vi "ReadSensorValues.vi"(10 "VISA resource name":refnum<visa-resource-name>, 11 "Sensor type":T1=enum."CAB 300-C SP3 (CAN)") -> ()   [LabVIEW 2012]
uses:
  <vilib>/nican/nicantsk.llb/CAN Interface.ctl
  SensorTypes.ctl
  SensorStates.ctl
  <vilib>/nican/nicantsk.llb/CAN Task Reference.ctl
  <vilib>/nican/nicantsk.llb/CAN Mode.ctl
  <vilib>/Analysis/3filter.llb/Filter Passband Type.ctl
  globalVariables.vi
  <vilib>/nican/nicantsk.llb/CAN Read Multi Chan Single Samp 1D Dbl.vi
  <vilib>/ptbypt/NI_PtbyPt.lvlib
  <vilib>/Analysis/NI_AALBase.lvlib
panel:
  out "Waveform Chart":dbl[](graph)
  out "Filtered current":dbl format="%.2f"
  in  "Cancel Measurement":bool
  out "new data":bool
  out "running":bool
  out "Sample number":i32
  in  "Interface":T2 items=["CAN0"=0, "CAN1"=1, "CAN2"=2, "CAN3"=3, "CAN4"=4, "CAN5"=5, "CAN6"=6, "CAN7"=7, "CAN8"=8, "CAN9"=9, "CAN10"=10, "CAN11"=11, "CAN12"=12, "CAN13"=13, "CAN14"=14, "CAN15"=15, "CAN16"=16, "CAN17"=17, "CAN18"=18, "CAN19"=19, "CAN20"=20, "CAN21"=21, "CAN22"=22, "CAN23"=23, "CAN24"=24, "CAN25"=25, "CAN26"=26, "CAN27"=27, "CAN28"=28, "CAN29"=29, "CAN30"=30, "CAN31"=31, "CAN32"=32, "CAN33"=33, "CAN34"=34, "CAN35"=35, "CAN36"=36, "CAN37"=37, "CAN38"=38, "CAN39"=39, "CAN40"=40, "CAN41"=41, "CAN42"=42, "CAN43"=43, "CAN44"=44, "CAN45"=45, "CAN46"=46, "CAN47"=47, "CAN48"=48, "CAN49"=49, "CAN50"=50, "CAN51"=51, "CAN52"=52, "CAN53"=53, "CAN54"=54, "CAN55"=55, "CAN56"=56, "CAN57"=57, "CAN58"=58, "CAN59"=59, "CAN60"=60, "CAN61"=61, "CAN62"=62, "CAN63"=63, "MAX default"=64, "CAN256 (Virtual)"=256, "CAN257 (Virtual)"=257]
  out "current":dbl format="%^#_5e"
  out "Error Flag":bool
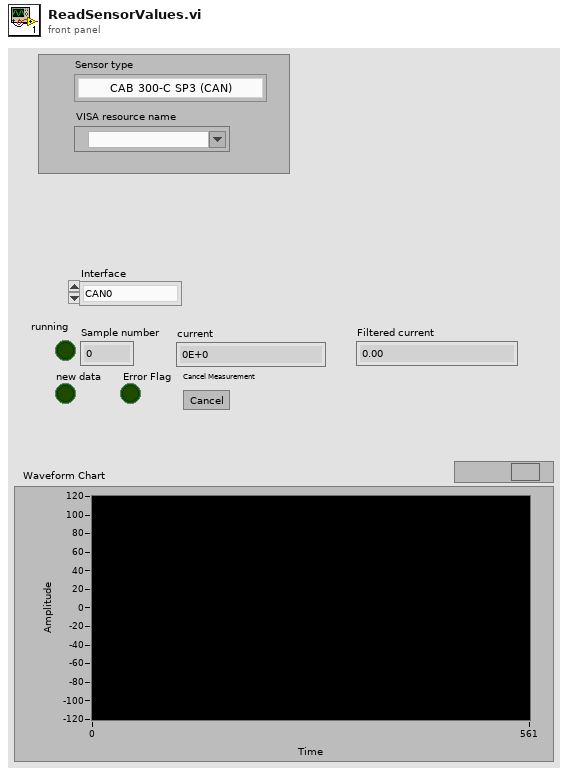
[diagram p1: front panel]
types:
  T1 = typedef "SensorTypes.ctl" = enum16{"ITL 900 (Analogue)", "CAB 300-C SP3 (CAN)", "xyz TODO (PWM)", "xyz TODO (LIN)", "xyz TODO (Analogue)"}
  T2 = typedef "CAN Interface.ctl" = u16
  T3 = typedef "SensorStates.ctl" = enum16{"init", "measure", "terminate"}
  T4 = typedef "CAN Task Reference.ctl" = u32
  T5 = typedef "NI_AALBase.lvlib/Filter Passband Type.ctl" = enum32{"Lowpass", "Highpass", "Bandpass", "Bandstop"}
  T6 = typedef "CAN Mode.ctl" = u16
  T7 = typedef "TimeValue.ctl" = cluster{"Time of measurement":timestamp, "Current value":dbl}
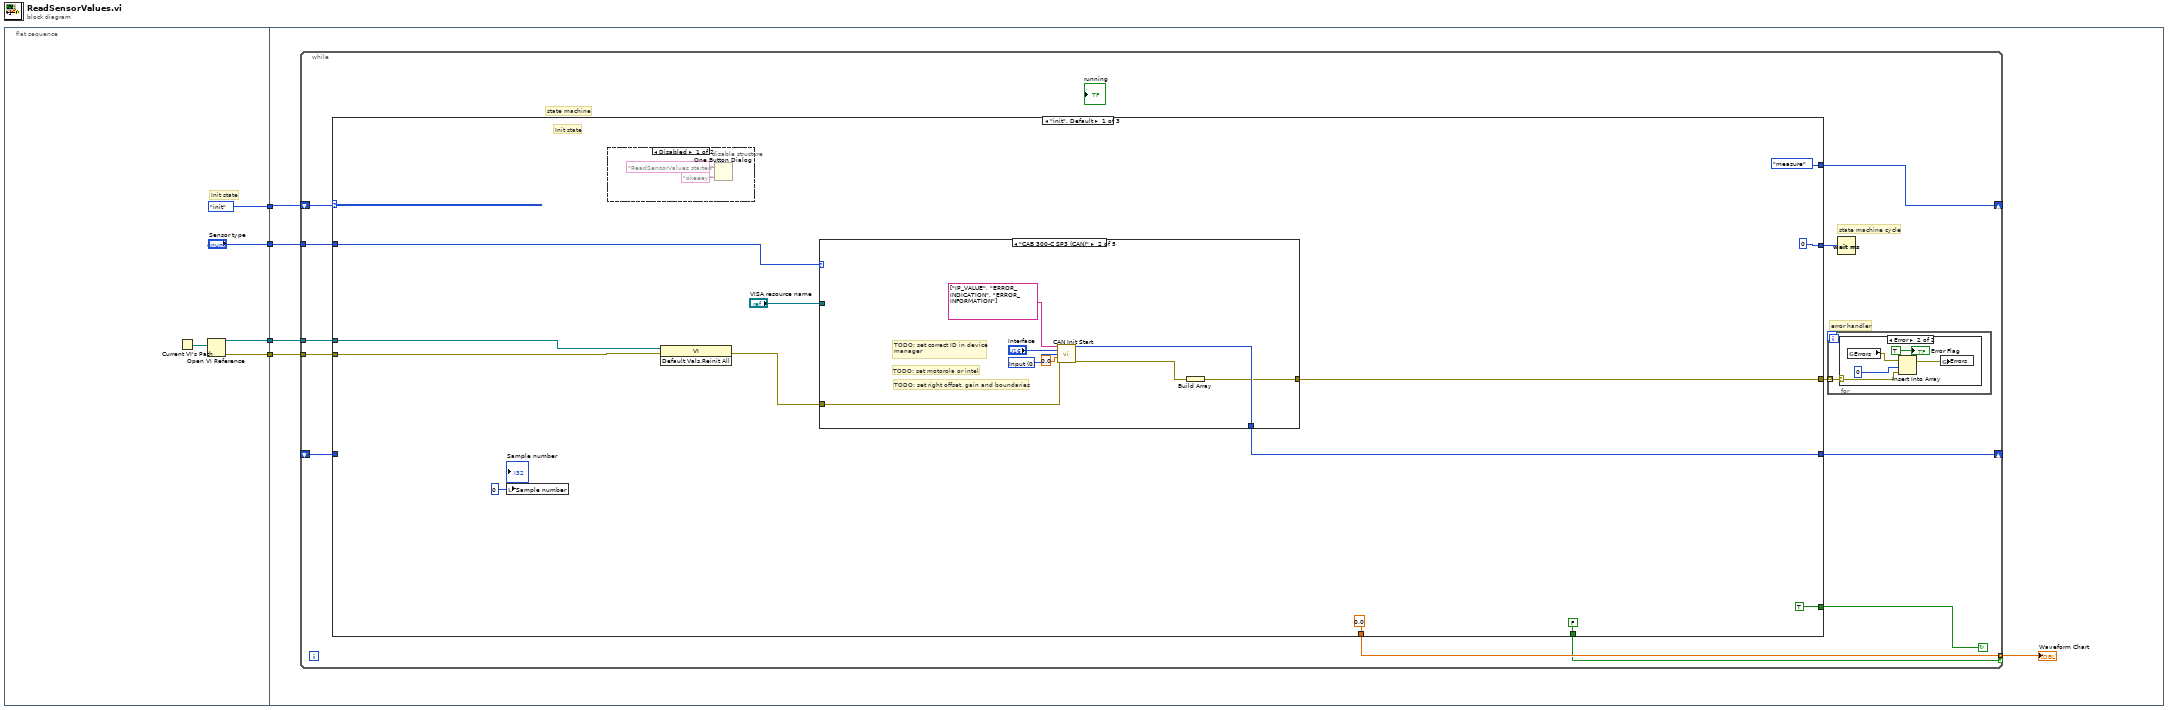
[diagram p0: block diagram]
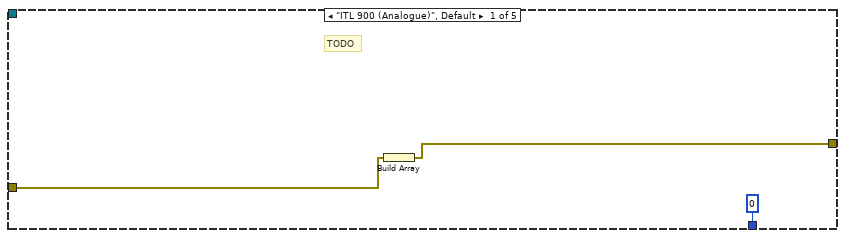
[diagram p4: hidden frame]
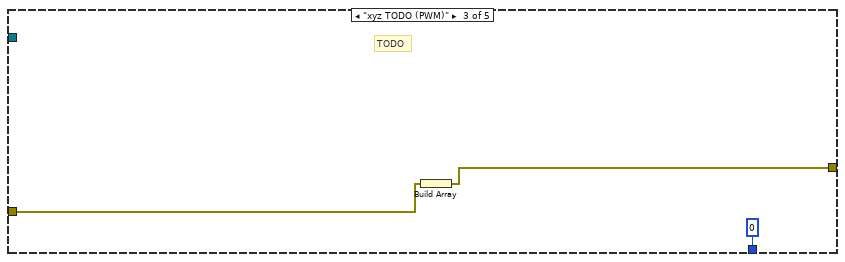
[diagram p5: hidden frame]
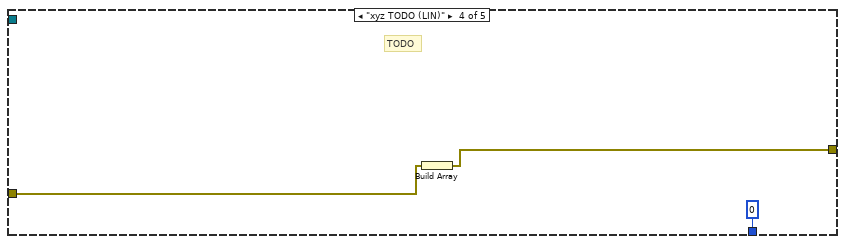
[diagram p6: hidden frame]
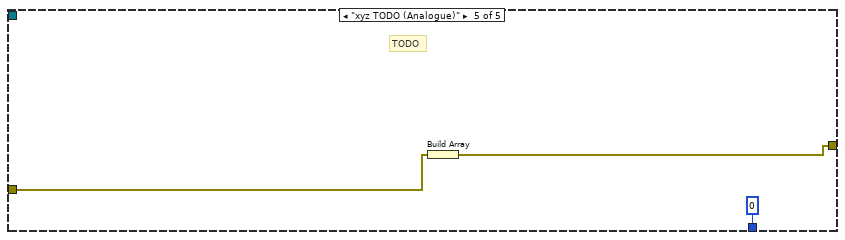
[diagram p7: hidden frame]
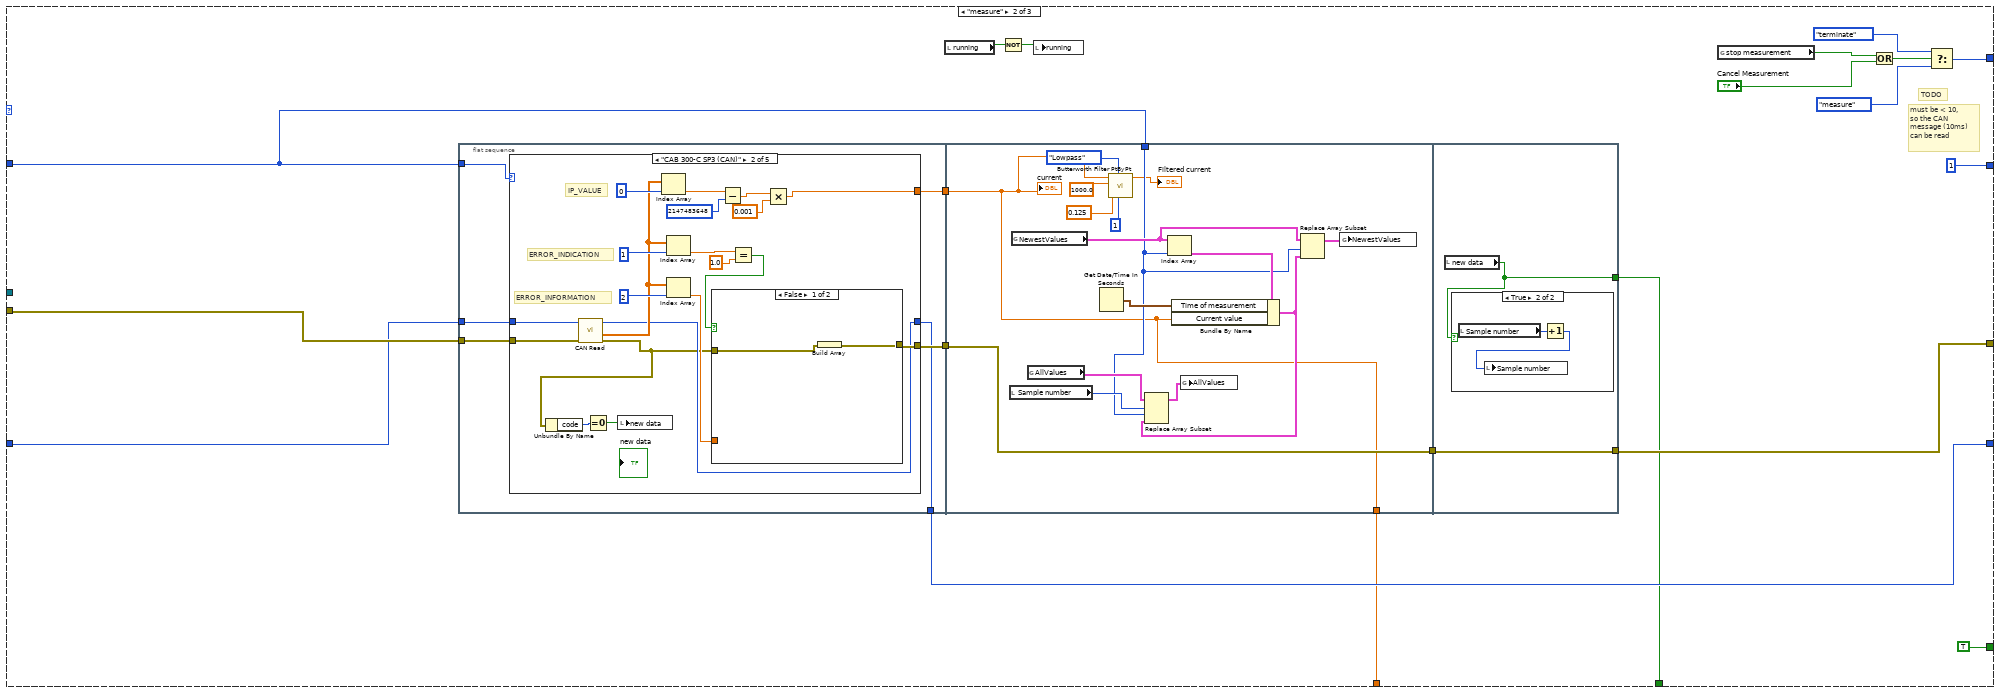
[diagram p8: hidden frame]
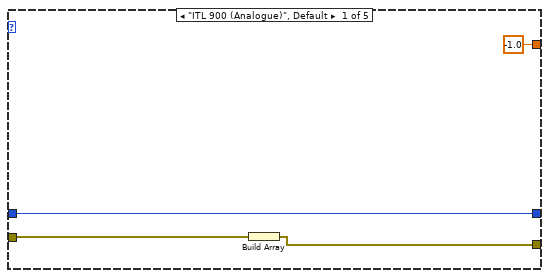
[diagram p9: hidden frame]
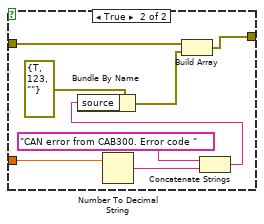
[diagram p10: hidden frame]
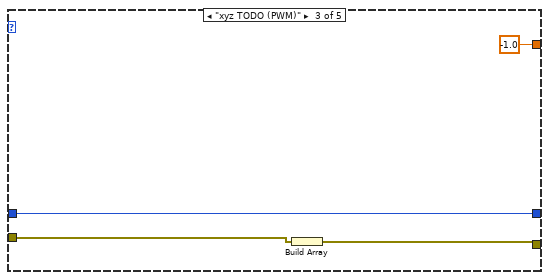
[diagram p11: hidden frame]
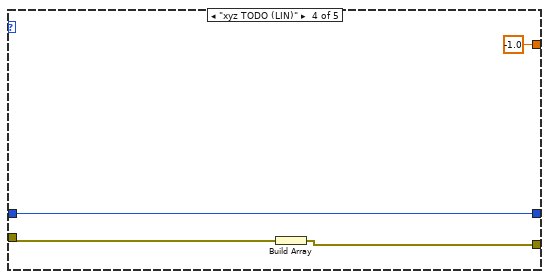
[diagram p12: hidden frame]
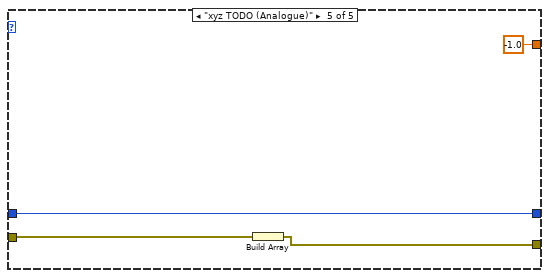
[diagram p13: hidden frame]
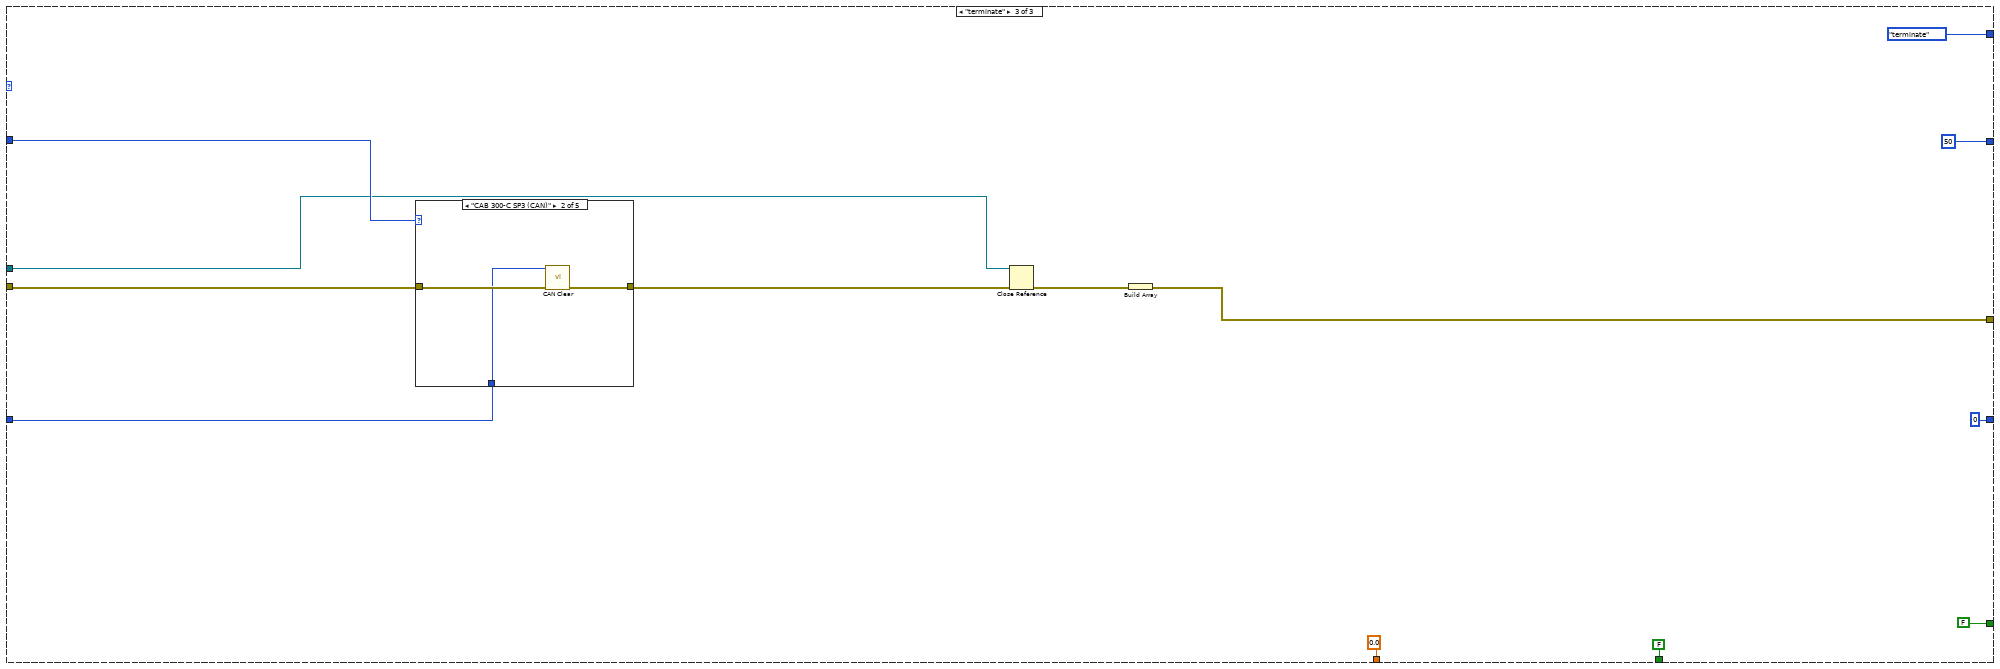
[diagram p15: hidden frame]
diagram:
  n1 = flat-sequence {
    tunnel: [SensorStates."init" ("States IEEE-488")] -> w4
    tunnel: [w9] -> w3
    tunnel: [w8] -> w2
    tunnel: ["Sensor type"] -> w1
    tunnel: w4 -> [w12]
    tunnel: w3 -> [w14]
    tunnel: w2 -> [w13]
    tunnel: w1 -> [w11]
    frame #0 {
      # "Init state"
      n2 = Current VI's Path() -> (path=w7:path)
      n3 = Open VI Reference(vi path=w7) -> (vi reference=w9:refnum<vi>, error out=w8:errorcluster)  [unwired: 2 in, 3 out]
    }
    frame #1 {
      n4 = while {
        tunnel: w14 -> [w25]
        tunnel: w13 -> [w24]
        shift-right: [w22] -> _
        shift-left: w12 -> [w23]
        shift-right: [w21] -> _
        shift-left: _ -> [w20]
        tunnel: w11 -> [w18]
        tunnel: [w16] -> w10 mode=indexing if=w15
        stop <- w17 continue-if-true
        # "state machine"
        # "error handler"
        # "state machine cycle"
        n5 = case shown="\"init\", Default" w23 {
          tunnel: [u32 0 ("milliseconds to wait") u32 1 ("milliseconds to wait") u32 50 ("milliseconds to wait")] -> w26
          tunnel: w25 -> [w43 _ w164]
          tunnel: w24 -> [w44 w83 w169]
          tunnel: [SensorStates."measure" ("States IEEE-488") w84 SensorStates."terminate" ("States IEEE-488")] -> w22
          tunnel: [w41 w73 T4 0 ("task reference out")] -> w21
          tunnel: w20 -> [_ w74 w168]
          tunnel: [w39 w75 w167] -> w19
          tunnel: w18 -> [w37 w79 w166]
          tunnel: [TRUE TRUE FALSE] -> w17
          tunnel: [0.0 ("Sample") w69 0.0 ("Sample")] -> w16
          tunnel: [FALSE ("new data") w68 FALSE ("new data")] -> w15
          frame "init", Default {
            # "Init state"
            n6 = local write "Sample number"(0 ("Sample number")) -> ()
            n7 = disable-structure shown="Disabled" {
              frame Disabled {
                n8 = One Button Dialog(message="ReadSensorValues started", button name ("OK")="okeeey!") -> ()  [unwired: 1 out]
              }
              frame Enabled {
              }
            }
            n9 = invoke class="VI" method="Default Vals.Reinit All"(reference=w43, error in=w44) -> (error out=w40:errorcluster)  [unwired: 1 in, 2 out]
            n10 = case shown="\"CAB 300-C SP3 (CAN)\"" w37 {
              tunnel: [T4 0 ("task reference out") w54 T4 0 ("task reference out") T4 0 ("task reference out") T4 0 ("task reference out")] -> w41
              tunnel: w40 -> [w50 w53 w60 w63 w67]
              tunnel: [w49 w51 w61 w64 w66] -> w39
              tunnel: "VISA resource name" -> [_ _ _ _ _]
              frame "ITL 900 (Analogue)", Default {
                # "TODO"
                n11 = Build Array(w50) -> (w49:errorcluster[])
              }
              frame "CAB 300-C SP3 (CAN)" {
                w55 = T6 0 items=["Input", "Output", "Timestamped Input", "Output Recent"] ("mode")
                # "TODO: set right offset, gain and boundaries"
                # "TODO: set motorola or intel"
                # "TODO: set correct ID in device\nmanager"
                n12 = call <vilib>:"CAN Init Start.vi"("channel list"=string[] ["IP_VALUE", "ERROR_INDICATION", "ERROR_INFORMATION"] ("Channel List"), "interface"="Interface", "mode"=w55, "sample rate"=0.0, "error in (no error)"=w53) -> ("task reference out"=w54:T4, "error out"=w52:errorcluster)  [unwired: 9 in]
                n13 = Build Array(w52) -> (w51:errorcluster[])
              }
              frame "xyz TODO (PWM)" {
                # "TODO"
                n14 = Build Array(w60) -> (w61:errorcluster[])
              }
              frame "xyz TODO (LIN)" {
                # "TODO"
                n15 = Build Array(w63) -> (w64:errorcluster[])
              }
              frame "xyz TODO (Analogue)" {
                # "TODO"
                n16 = Build Array(w67) -> (w66:errorcluster[])
              }
            }
          }
          frame "measure" {
            # "TODO"
            # "must be < 10,\nso the CAN \nmessage (10ms) \ncan be read"
            n17 = flat-sequence {
              tunnel: [w92] -> w82
              tunnel: [w91] -> w81
              tunnel: w83 -> [w93]
              tunnel: w79 -> [w90]
              tunnel: w74 -> [w89]
              tunnel: [w88] -> w73
              tunnel: w82 -> [w152]
              tunnel: w81 -> [w140]
              tunnel: [w152] -> w80
              tunnel: w79 -> [w148]
              tunnel: [w140] -> w69
              tunnel: w80 -> [w157]
              tunnel: [w157] -> w75
              tunnel: [w156] -> w68
              frame #0 {
                n18 = case shown="\"CAB 300-C SP3 (CAN)\"" w90 {
                  tunnel: w93 -> [w95 w117 w129 w134 w137]
                  tunnel: [w96 w111 w130 w135 w138] -> w92
                  tunnel: [-1.0 ("Sample") w98 -1.0 ("Sample") -1.0 ("Sample") -1.0 ("Sample")] -> w91
                  tunnel: w89 -> [w94 w107 w128 w132 w136]
                  tunnel: [w94 w106 w128 w132 w136] -> w88
                  frame "ITL 900 (Analogue)", Default {
                    n19 = Build Array(w95) -> (w96:errorcluster[])
                  }
                  frame "CAB 300-C SP3 (CAN)" {
                    # "ERROR_INFORMATION"
                    # "ERROR_INDICATION"
                    # "IP_VALUE"
                    n20 = call-poly <vilib>:"CAN Read.vi"("error in (no error)"=w117, "task reference in"=w107) -> ("error out"=w105:errorcluster, "multi-chan single-samp 1D dbl"=w110:dbl[], "task reference out"=w106:T4)  [unwired: 6 in, 1 out]
                    n21 = Unbundle By Name(w105) -> ("code"=w104:i32)
                    n22 = Equal To 0?(x=w104) -> (x = 0?=w103:bool)
                    n23 = local write "new data"(w103) -> ()
                    n24 = Index Array(array=w110, index=0) -> (element=w102:dbl)
                    n25 = Index Array(array=w110, index=1) -> (element=w113:dbl)
                    n26 = Index Array(array=w110, index=2) -> (element=w109:dbl)
                    n27 = Subtract(x=w102, y=u32 2147483648) -> (x-y=w100:dbl)
                    n28 = Equal?(x=w113, y=1.0) -> (x = y?=w108:bool)
                    n29 = case shown="False" w108 {
                      tunnel: w105 -> [w119 w127]
                      tunnel: [w118 w126] -> w111
                      tunnel: w109 -> [_ w121]
                      frame False {
                        n30 = Build Array(w119) -> (w118:errorcluster[])
                      }
                      frame True {
                        n31 = Number To Decimal String(number=w121) -> (decimal integer string=w122:string)  [unwired: 1 in]
                        n32 = Concatenate Strings("CAN error from CAB300. Error code ", w122) -> (w120:string)
                        n33 = Bundle By Name(cluster=errorcluster {"status"=TRUE, "code"=123, "source"=""} ("error out"), "source"=w120) -> (w124:errorcluster)
                        n34 = Build Array(w127, w124) -> (w126:errorcluster[])
                      }
                    }
                    n35 = Multiply(x=w100, y=0.001) -> (x*y=w98:dbl)
                  }
                  frame "xyz TODO (PWM)" {
                    n36 = Build Array(w129) -> (w130:errorcluster[])
                  }
                  frame "xyz TODO (LIN)" {
                    n37 = Build Array(w134) -> (w135:errorcluster[])
                  }
                  frame "xyz TODO (Analogue)" {
                    n38 = Build Array(w137) -> (w138:errorcluster[])
                  }
                }
              }
              frame #1 {
                n39 = local read "Sample number"() -> (w149:i32)
                n40 = global read "globalVariables.vi" "NewestValues"() -> (w153:T7[])
                n41 = global read "globalVariables.vi" "AllValues"() -> (w150:T7[][])
                n42 = Get Date/Time In Seconds() -> (seconds since 1Jan1904=w154:timestamp)
                n43 = call <vilib>:"Butterworth Filter PtByPt.vi"("order"=1, "filter type"=Filter_Passband_Type."Lowpass", "low cutoff freq: fl"=0.125, "sampling freq: fs"=1000.0, "x"=w140) -> ("Filtered x"=→"Filtered current":dbl)  [unwired: 4 in, 1 out]
                n44 = Index Array(array=w153, index=w148) -> (element=w155:T7)
                n45 = Bundle By Name(cluster=w155, "Time of measurement"=w154, "Current value"=w140) -> (w147:T7)
                n46 = Replace Array Subset(array=w150, new element=w147, index (row)=w149, index (col)=w148) -> (w146:T7[][])
                n47 = global write "globalVariables.vi" "AllValues"(w146) -> ()
                n48 = Replace Array Subset(array=w153, new element=w147, index=w148) -> (w151:T7[])
                n49 = global write "globalVariables.vi" "NewestValues"(w151) -> ()
                "current" <- w140
              }
              frame #2 {
                n50 = local read "new data"() -> (w156:bool)
                n51 = case shown="True" w156 {
                  frame False {
                  }
                  frame True {
                    n52 = local read "Sample number"() -> (w159:i32)
                    n53 = Increment(x=w159) -> (x+1=w158:i32)
                    n54 = local write "Sample number"(w158) -> ()
                  }
                }
              }
            }
            n55 = local read "running"() -> (w77:bool)
            n56 = Not(x=w77) -> (.not. x?=w78:bool)
            n57 = local write "running"(w78) -> ()
            n58 = global read "globalVariables.vi" "stop measurement"() -> (w72:bool)
            n59 = Or(x=w72, y="Cancel Measurement") -> (x .or. y?=w70:bool)
            n60 = Select(t=SensorStates."terminate" ("States IEEE-488"), s=w70, f=SensorStates."measure" ("States IEEE-488")) -> (s? t:f=w84:T3)
          }
          frame "terminate" {
            n61 = case shown="\"CAB 300-C SP3 (CAN)\"" w166 {
              tunnel: w169 -> [w173 w176 w177 w178 w179]
              tunnel: [w173 w175 w177 w178 w179] -> w163
              tunnel: w168 -> [_ w174 _ _ _]
              frame "ITL 900 (Analogue)", Default {
              }
              frame "CAB 300-C SP3 (CAN)" {
                n62 = call <vilib>:"CAN Clear.vi"("error in (no error)"=w176, "task reference in"=w174) -> ("error out"=w175:errorcluster)  [unwired: 9 in]
              }
              frame "xyz TODO (PWM)" {
              }
              frame "xyz TODO (LIN)" {
              }
              frame "xyz TODO (Analogue)" {
              }
            }
            n63 = Close Reference(reference=w164, error in (no error)=w163) -> (error out=w171:errorcluster)
            n64 = Build Array(w171) -> (w167:errorcluster[])
          }
        }
        n65 = for {
          tunnel: w19 -> [w27] mode=indexing
          n66 = case shown="Error" w27 {
            selector: w27 -> [_ w31]
            frame No Error {
            }
            frame Error {
              n67 = global read "globalVariables.vi" "Errors"() -> (w29:errorcluster[])
              n68 = Insert Into Array(array=w29, index=0, new element=w31) -> (w28:errorcluster[])
              n69 = global write "globalVariables.vi" "Errors"(w28) -> ()
              "Error Flag" <- TRUE ("Error Flag")
            }
          }
        }
        n70 = Wait (ms)(milliseconds to wait=w26) -> ()  [unwired: 1 out]
      }
      "Waveform Chart" <- w10
    }
  }
